vi "RequestFGV.vi"(7 "Actions":T1, 8 "error in (no error)":errorcluster, 9 "Data In":string, 10 "RUID":string) -> (0 "error out":errorcluster, 1 "Data Out":string)   [LabVIEW 2015]
uses:
  TypeDef/RequestActionEnum.ctl
  TypeDef/RequestStateCluster.ctl
  LVClasses/Request/Request.lvclass
  TypeDef/Limits.ctl
  LVClasses/Request/Request.lvclass/Request.ctl
  LVClasses/Request/Read Room Number.vi
  LVClasses/Request/Write AckName.vi
  LVClasses/Request/Write AckTime.vi
  LVClasses/Request/Read RequestID.vi
  LVClasses/Request/Write FulfilledName.vi
  LVClasses/Request/Write FulfilledTime.vi
  <vilib>/Utility/error.llb/Error Cluster From Error Code.vi
  <vilib>/ErrorRing/Error Ring.xnode
  TypeDef/PersonnelAndTime.ctl
  Database/DatabaseApi.lvlib
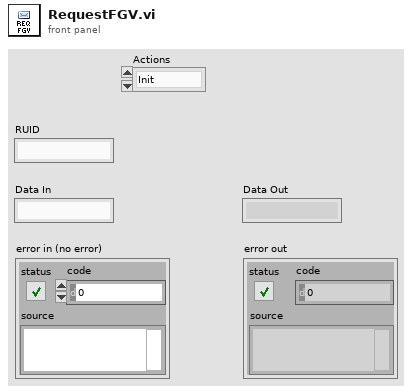
[diagram p1: front panel]
types:
  T1 = typedef "RequestActionEnum.ctl" = enum16{"Init", "ReadRequests", "ReadRequest", "AddRequest", "RemoveRequest", "ToDisk", "Ack", "Complete", "CheckAlarms", "PIntoRoom", "Read Summary", "GetRequestForRoom"}
  T2 = typedef "Limits.ctl" = cluster{"AckLimit":dbl, "CompleteLimit":dbl}
  T3 = typedef "RequestStateCluster.ctl" = cluster{"Requests":refnum<class "Request.lvclass">[], "Limits":cluster{"AckLimit":dbl, "CompleteLimit":dbl}}
  T4 = typedef "PersonnelAndTime.ctl" = cluster{"Personnel":string, "TimeStamp":string}
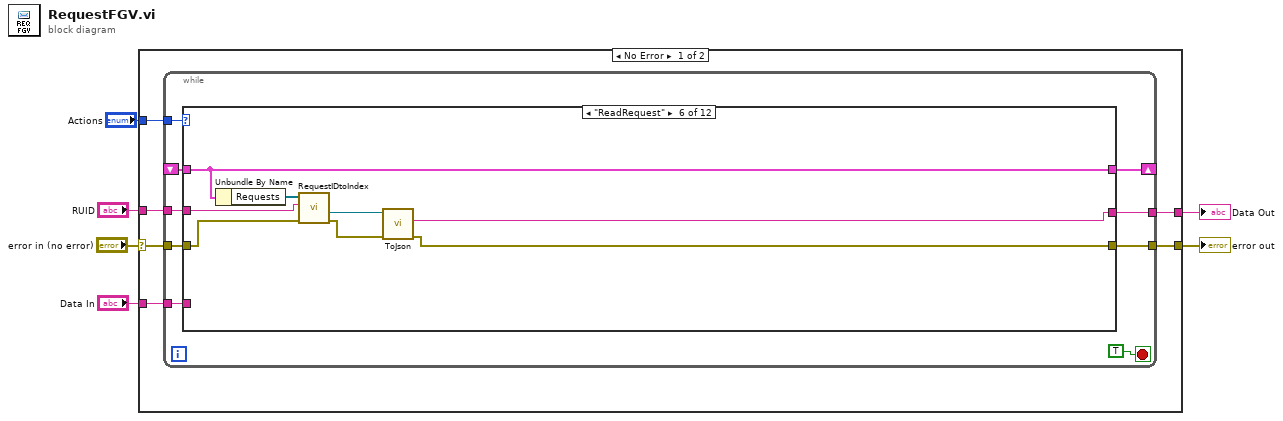
[diagram p0: block diagram]
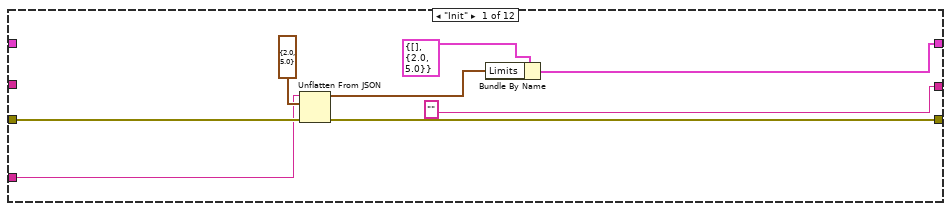
[diagram p2: hidden frame]
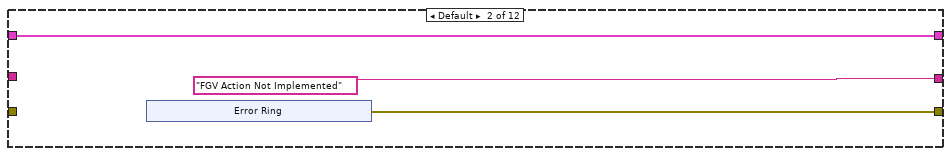
[diagram p3: hidden frame]
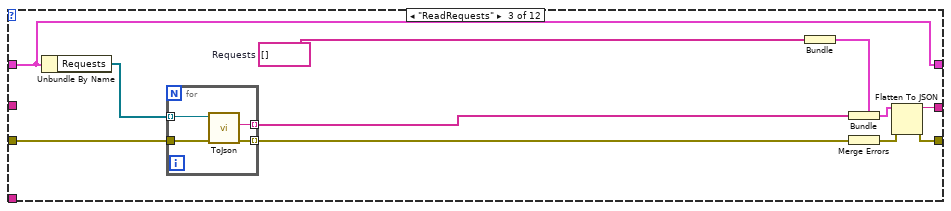
[diagram p4: hidden frame]
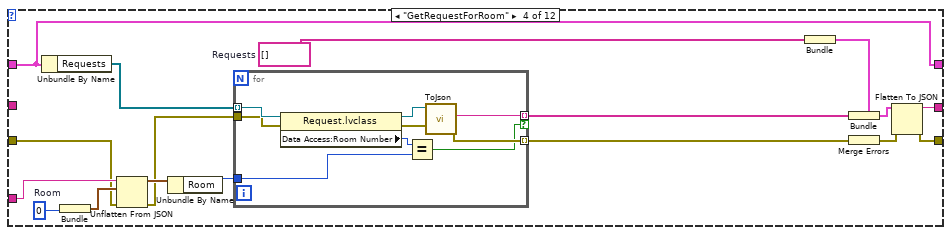
[diagram p5: hidden frame]
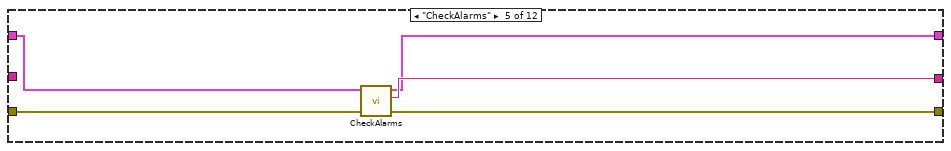
[diagram p6: hidden frame]
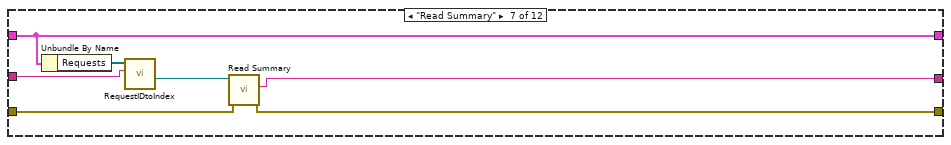
[diagram p7: hidden frame]
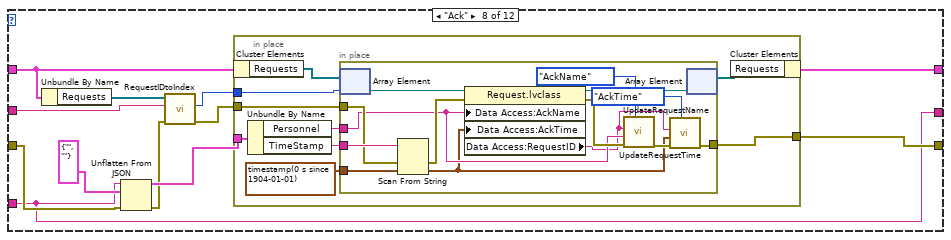
[diagram p8: hidden frame]
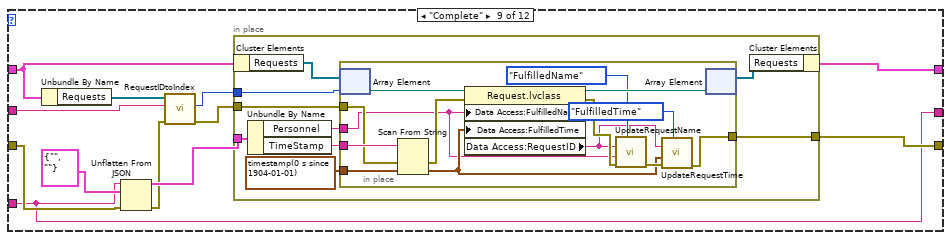
[diagram p9: hidden frame]
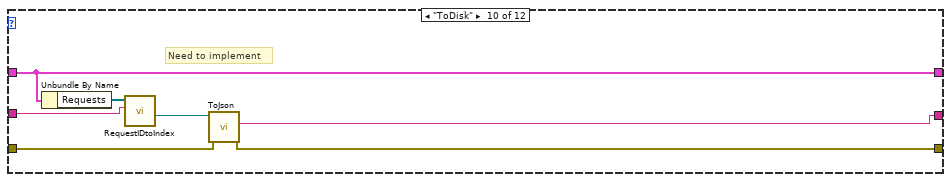
[diagram p10: hidden frame]
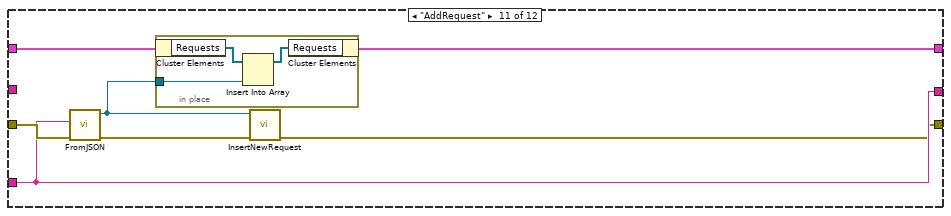
[diagram p11: hidden frame]
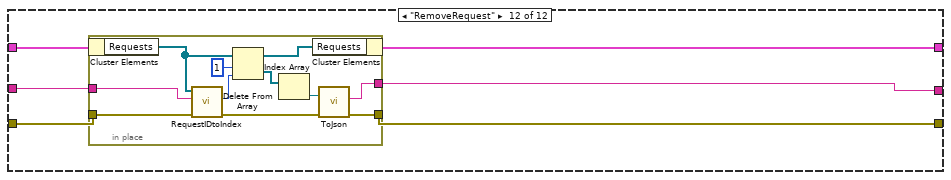
[diagram p12: hidden frame]
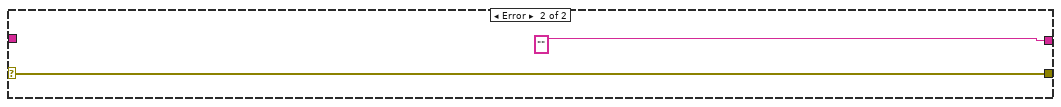
[diagram p13: hidden frame]
diagram:
  n1 = case shown="No Error" "error in (no error)" {
    selector: "error in (no error)" -> [w8 w203]
    tunnel: [w7 w203] -> w5
    tunnel: "Actions" -> [w12 _]
    tunnel: "Data In" -> [w11 _]
    tunnel: [w10 "" ("Data In")] -> w2
    tunnel: "RUID" -> [w9 _]
    frame No Error {
      n2 = while {
        shift-right: [w17] -> _
        shift-left: _ -> [w16]
        tunnel: w12 -> [w20]
        tunnel: w11 -> [w19]
        tunnel: [w18] -> w10
        tunnel: w9 -> [w15]
        tunnel: w8 -> [w14]
        tunnel: [w13] -> w7
        stop <- TRUE stop-if-true
        n3 = case shown="\"ReadRequest\"" w20 {
          tunnel: w19 -> [w25 _ _ w57 _ _ _ w103 w138 _ w179 _]
          tunnel: ["" ("Data In") "FGV Action Not Implemented" ("Data In") w45 w66 w81 w87 w94 w103 w138 w171 w179 w186] -> w18
          tunnel: [w23 w30 w44 w65 w79 w89 w96 w102 w137 w173 w181 w190] -> w17
          tunnel: w16 -> [_ w30 w44 w65 w80 w89 w96 w107 w142 w173 w182 w191]
          tunnel: w15 -> [_ _ _ _ _ w90 w97 w109 w144 w174 _ w189]
          tunnel: w14 -> [w28 _ w41 w54 w83 w85 w92 w106 w141 w169 w180 w188]
          tunnel: [w27 w32 w40 w62 w82 w86 w93 w105 w140 w170 w176 w187] -> w13
          frame "Init" {
            n4 = Unflatten From JSON(JSON string=w25, type and defaults=T2 {"AckLimit"=2.0, "CompleteLimit"=5.0} ("Limits"), error in (no error)=w28) -> (value=w22:T2, error out=w27:errorcluster)  [unwired: 4 in]
            n5 = Bundle By Name(cluster=T3 {"Requests"=[], "Limits"={"AckLimit"=2.0, "CompleteLimit"=5.0}} ("Cluster"), "Limits"=w22) -> (w23:T3)
          }
          frame Default {
            n6 = xnode "Error Ring"() -> ("error out"=w32:errorcluster)
          }
          frame "ReadRequests" {
            w47 = string[] []  # Requests
            n7 = Unbundle By Name(w44) -> ("Requests"=w43:refnum<class "Request.lvclass">[])
            n8 = for {
              tunnel: w43 -> [w52] mode=indexing
              tunnel: [w51] -> w42 mode=indexing
              tunnel: w41 -> [w50]
              tunnel: [w49] -> w39 mode=indexing
              n9 = call "ToJson.vi"("error in (no error)"=w50, "Request"=w52) -> ("error out"=w49:errorcluster, "Request"=w51:string)  [unwired: 8 in]
            }
            n10 = Bundle("Requests"=w47) -> (w48:cluster{"Requests":string[]})  [unwired: 1 in]
            n11 = Bundle(cluster=w48, "Requests"=w42) -> (w46:cluster{"Requests":string[]})
            n12 = Merge Errors(w39) -> (w38:errorcluster)
            n13 = Flatten To JSON(anything=w46, error in (no error)=w38) -> (JSON string=w45:string, 11:w40:errorcluster)  [unwired: 1 in]
          }
          frame "GetRequestForRoom" {
            w59 = 0  # Room
            w68 = string[] []  # Requests
            n14 = Unbundle By Name(w65) -> ("Requests"=w64:refnum<class "Request.lvclass">[])
            n15 = Bundle("Room"=w59) -> (w58:cluster{"Room":i32})  [unwired: 1 in]
            n16 = Unflatten From JSON(JSON string=w57, type and defaults=w58, error in (no error)=w54) -> (value=w56:cluster{"Room":i32}, error out=w53:errorcluster)  [unwired: 4 in]
            n17 = Unbundle By Name(w56) -> ("Room"=w55:i32)
            n18 = for {
              tunnel: w64 -> [w78] mode=indexing
              tunnel: [w74] -> w63 mode=indexing if=w70
              tunnel: w53 -> [w77]
              tunnel: [w75] -> w61 mode=indexing
              tunnel: w55 -> [w71]
              n19 = property class="Request.lvclass"(reference=w78, error in=w77) -> (reference out=w73:refnum<class "Request.lvclass">, error out=w76:errorcluster, "Data Access:Room Number"=w72:i32)
              n20 = Equal?(x=w72, y=w71) -> (x = y?=w70:bool)
              n21 = call "ToJson.vi"("error in (no error)"=w76, "Request"=w73) -> ("error out"=w75:errorcluster, "Request"=w74:string)  [unwired: 8 in]
            }
            n22 = Bundle("Requests"=w68) -> (w69:cluster{"Requests":string[]})  [unwired: 1 in]
            n23 = Bundle(cluster=w69, "Requests"=w63) -> (w67:cluster{"Requests":string[]})
            n24 = Merge Errors(w61) -> (w60:errorcluster)
            n25 = Flatten To JSON(anything=w67, error in (no error)=w60) -> (JSON string=w66:string, 11:w62:errorcluster)  [unwired: 1 in]
          }
          frame "CheckAlarms" {
            n26 = call "CheckAlarms.vi"("error in (no error)"=w83, "Cluster"=w80) -> ("error out"=w82:errorcluster, "JSON string"=w81:string, "Requests Out"=w79:T3)  [unwired: 7 in]
          }
          frame "ReadRequest" {
            n27 = Unbundle By Name(w89) -> ("Requests"=w91:refnum<class "Request.lvclass">[])
            n28 = call "RequestIDtoIndex.vi"("error in (no error)"=w85, "RUID"=w90, "REquest In"=w91) -> ("error out"=w84:errorcluster, "Request"=w88:refnum<class "Request.lvclass">)  [unwired: 5 in, 2 out]
            n29 = call "ToJson.vi"("error in (no error)"=w84, "Request"=w88) -> ("error out"=w86:errorcluster, "Request"=w87:string)  [unwired: 8 in]
          }
          frame "Read Summary" {
            n30 = Unbundle By Name(w96) -> ("Requests"=w98:refnum<class "Request.lvclass">[])
            n31 = call "RequestIDtoIndex.vi"("RUID"=w97, "REquest In"=w98) -> ("Request"=w95:refnum<class "Request.lvclass">)  [unwired: 6 in, 3 out]
            n32 = call "Read Summary.vi"("error in (no error)"=w92, "Request in"=w95) -> ("error out"=w93:errorcluster, "Description"=w94:string)  [unwired: 7 in, 1 out]
          }
          frame "Ack" {
            n33 = Unbundle By Name(w107) -> ("Requests"=w110:refnum<class "Request.lvclass">[])
            n34 = Unflatten From JSON(JSON string=w103, type and defaults=T4 {"Personnel"="", "TimeStamp"=""}, error in (no error)=w106) -> (value=w104:T4, error out=w100:errorcluster)  [unwired: 4 in]
            n35 = call "RequestIDtoIndex.vi"("error in (no error)"=w100, "RUID"=w109, "REquest In"=w110) -> ("error out"=w99:errorcluster, "Index"=w101:i32)  [unwired: 5 in, 2 out]
            n36 = in-place {
              in-place-border: w99 -> [w117]
              in-place-border: [w116] -> w105
              in-place-border: w104 -> [w115]
              in-place-border: w101 -> [w111]
              n37 = in-place-cluster #1(w107) -> ("Requests"=w119:refnum<class "Request.lvclass">[])
              n38 = Unbundle By Name(w115) -> ("Personnel"=w114:string, "TimeStamp"=w113:string)
              n39 = in-place {
                in-place-border: w117 -> [w129]
                in-place-border: [w123] -> w116
                in-place-border: w114 -> [w125]
                in-place-border: w113 -> [w131]
                in-place-border: timestamp(0 s since 1904-01-01) ("AckTime") -> [w130]
                n40 = in-place-array #2(w119, w111) -> (w133:refnum<class "Request.lvclass">)
                n41 = Scan From String(input string=w131, error in=w129, default 1=w130) -> (error out=w128:errorcluster, output 1=w120:timestamp)  [unwired: 2 in, 2 out]
                n42 = property class="Request.lvclass"(reference=w133, error in=w128, "Data Access:AckName"=w125, "Data Access:AckTime"=w120) -> (reference out=w132:refnum<class "Request.lvclass">, error out=w127:errorcluster, "Data Access:RequestID"=w122:string)
                n43 = call "UpdateRequestName.vi"("NameType"=enum16{"StartName", "AckName", "FulfilledName"}."AckName", "error in"=w127, "Name"=w125, "RequestID"=w122) -> ("error out"=w124:errorcluster)  [unwired: 7 in]
                n44 = call "UpdateRequestTime.vi"("TimeType"=enum16{"StartTime", "AckTime", "FulfilledTime"}."AckTime", "error in"=w124, "Time"=w120, "RequestID"=w122) -> ("error out"=w123:errorcluster)  [unwired: 7 in]
                n45 = in-place-array #2(w132) -> (w118:refnum<class "Request.lvclass">[])  [unwired: 1 out]
              }
              n46 = in-place-cluster #1("Requests"=w118) -> (w102:T3)
            }
          }
          frame "Complete" {
            n47 = Unbundle By Name(w142) -> ("Requests"=w145:refnum<class "Request.lvclass">[])
            n48 = Unflatten From JSON(JSON string=w138, type and defaults=T4 {"Personnel"="", "TimeStamp"=""}, error in (no error)=w141) -> (value=w139:T4, error out=w135:errorcluster)  [unwired: 4 in]
            n49 = call "RequestIDtoIndex.vi"("error in (no error)"=w135, "RUID"=w144, "REquest In"=w145) -> ("error out"=w134:errorcluster, "Index"=w136:i32)  [unwired: 5 in, 2 out]
            n50 = in-place {
              in-place-border: w134 -> [w152]
              in-place-border: [w151] -> w140
              in-place-border: w139 -> [w150]
              in-place-border: w136 -> [w146]
              n51 = in-place-cluster #3(w142) -> ("Requests"=w154:refnum<class "Request.lvclass">[])
              n52 = Unbundle By Name(w150) -> ("Personnel"=w149:string, "TimeStamp"=w148:string)
              n53 = in-place {
                in-place-border: w152 -> [w164]
                in-place-border: [w160] -> w151
                in-place-border: w149 -> [w156]
                in-place-border: w148 -> [w166]
                in-place-border: timestamp(0 s since 1904-01-01) ("AckTime") -> [w165]
                n54 = in-place-array #4(w154, w146) -> (w168:refnum<class "Request.lvclass">)
                n55 = Scan From String(input string=w166, error in=w164, default 1=w165) -> (error out=w163:errorcluster, output 1=w157:timestamp)  [unwired: 2 in, 2 out]
                n56 = property class="Request.lvclass"(reference=w168, error in=w163, "Data Access:FulfilledName"=w156, "Data Access:FulfilledTime"=w157) -> (reference out=w167:refnum<class "Request.lvclass">, error out=w162:errorcluster, "Data Access:RequestID"=w155:string)
                n57 = call "UpdateRequestName.vi"("NameType"=enum16{"StartName", "AckName", "FulfilledName"}."FulfilledName", "error in"=w162, "Name"=w156, "RequestID"=w155) -> ("error out"=w161:errorcluster)  [unwired: 7 in]
                n58 = call "UpdateRequestTime.vi"("TimeType"=enum16{"StartTime", "AckTime", "FulfilledTime"}."FulfilledTime", "error in"=w161, "Time"=w157, "RequestID"=w155) -> ("error out"=w160:errorcluster)  [unwired: 7 in]
                n59 = in-place-array #4(w167) -> (w153:refnum<class "Request.lvclass">[])  [unwired: 1 out]
              }
              n60 = in-place-cluster #3("Requests"=w153) -> (w137:T3)
            }
          }
          frame "ToDisk" {
            # "Need to implement"
            n61 = Unbundle By Name(w173) -> ("Requests"=w175:refnum<class "Request.lvclass">[])
            n62 = call "RequestIDtoIndex.vi"("RUID"=w174, "REquest In"=w175) -> ("Request"=w172:refnum<class "Request.lvclass">)  [unwired: 6 in, 3 out]
            n63 = call "ToJson.vi"("error in (no error)"=w169, "Request"=w172) -> ("error out"=w170:errorcluster, "Request"=w171:string)  [unwired: 8 in]
          }
          frame "AddRequest" {
            n64 = call "FromJSON.vi"("error in (no error)"=w180, "Request"=w179) -> ("error out"=w178:errorcluster, "Request out"=w177:refnum<class "Request.lvclass">)  [unwired: 8 in]
            n65 = in-place {
              in-place-border: w177 -> [w183]
              n66 = in-place-cluster #5(w182) -> ("Requests"=w185:refnum<class "Request.lvclass">[])
              n67 = Insert Into Array(array=w185, new element=w183) -> (w184:refnum<class "Request.lvclass">[])  [unwired: 1 in]
              n68 = in-place-cluster #5("Requests"=w184) -> (w181:T3)
            }
            n69 = call "InsertNewRequest.vi"("error in"=w178, "Request.lvclass"=w177) -> ("error out"=w176:errorcluster)  [unwired: 8 in, 1 out]
          }
          frame "RemoveRequest" {
            n70 = in-place {
              in-place-border: w189 -> [w200]
              in-place-border: w188 -> [w196]
              in-place-border: [w195] -> w187
              in-place-border: [w194] -> w186
              n71 = in-place-cluster #6(w191) -> ("Requests"=w201:refnum<class "Request.lvclass">[])
              n72 = call "RequestIDtoIndex.vi"("error in (no error)"=w196, "RUID"=w200, "REquest In"=w201) -> ("error out"=w197:errorcluster, "Index"=w193:i32)  [unwired: 5 in, 2 out]
              n73 = Delete From Array(array=w201, length=1, index=w193) -> (deleted portion=w199:refnum<class "Request.lvclass">[], array with subset deleted=w202:refnum<class "Request.lvclass">[])
              n74 = Index Array(array=w199) -> (element=w198:refnum<class "Request.lvclass">)  [unwired: 1 in]
              n75 = in-place-cluster #6("Requests"=w202) -> (w190:T3)
              n76 = call "ToJson.vi"("error in (no error)"=w197, "Request"=w198) -> ("error out"=w195:errorcluster, "Request"=w194:string)  [unwired: 8 in]
            }
          }
        }
      }
    }
    frame Error {
    }
  }
  "Data Out" <- w2
  "error out" <- w5
